vi "Check Mouse.vi"(7 "Packed refs":T1, 8 "error in (no error)":errorcluster, 11 "Board Game in":refnum<class "Board Game.lvclass">) -> (0 "error out":errorcluster, 3 "Board Game out":refnum<class "Board Game.lvclass">)   [LabVIEW 2021, in "Board Game.lvclass"]
uses:
  Board Game.lvclass
  Application/Packed Refs.ctl
  GameEl_class/private/Enum Direction.ctl
  LVApp/Modules/Sound Manager/Typedefs/Sound Effects.ctl
  Board Game.lvclass/Board Game.ctl
  GameEl_class/GameEl.lvclass/GameEl.ctl
  Mouse/Mouse.lvclass/Mouse.ctl
  <vilib>/numeric/Random Number (Range) U64.vi
  GameEl_class/Write Visible.vi
  Mouse/Write Init Mouse.vi
  Snake_class/Read Snake Head.vi
  GameEl_class/Read Visible.vi
  GameEl_class/Read position.vi
  <vilib>/numeric/sub_Random U32.vi
  Mouse/Mouse.lvclass
  C:/Users/poche/Programs/LabVIEW/imposible snake/GameEl_class/GameEl.lvclass
  Snake_class/Snake.lvclass
  GameEl_class/GameEl.lvclass
  Application/Application.lvclass
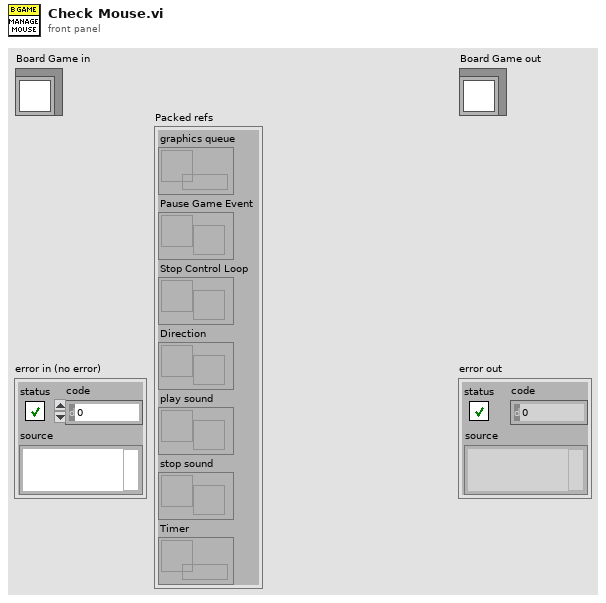
[diagram p1: front panel]
types:
  T1 = typedef "Application.lvclass/Packed Refs.ctl" = cluster{"graphics queue":refnum<queue>, "Pause Game Event":refnum<user-event>, "Stop Control Loop":refnum<user-event>, "Direction":refnum<notifier>, "play sound":refnum<user-event>, "stop sound":refnum<user-event>, "Timer":refnum<data-value>}
  T2 = typedef "Sound Effects.ctl" = enum16{"Bomb In", "Bomb Out", "Bomb Touched", "Game Over", "Victory", "Eat", "10 Fruits", "Eat2", "Eat3", "Eat4", "MaxShield", "Shield", "10p", "Grape In", "Grape Out", "20p", "30p", "40p", "50p", "60p", "70p", "80p", "90p", "100p", "All shields cracked", "Mouse In", "Mouse Out", "Mouse Eaten", "Grape Eaten", "States Recover", "Broken Shield", "Bonus", "Happy Time", "explode", "Game over musica", "Back Music", "Shield Catch", "Evil lough", "Cricket In", "Cricket eaten", "Lets Go", "Jump1", "Jump2", "Jump3", "Unstoppable", "Troll Music", "winner"}
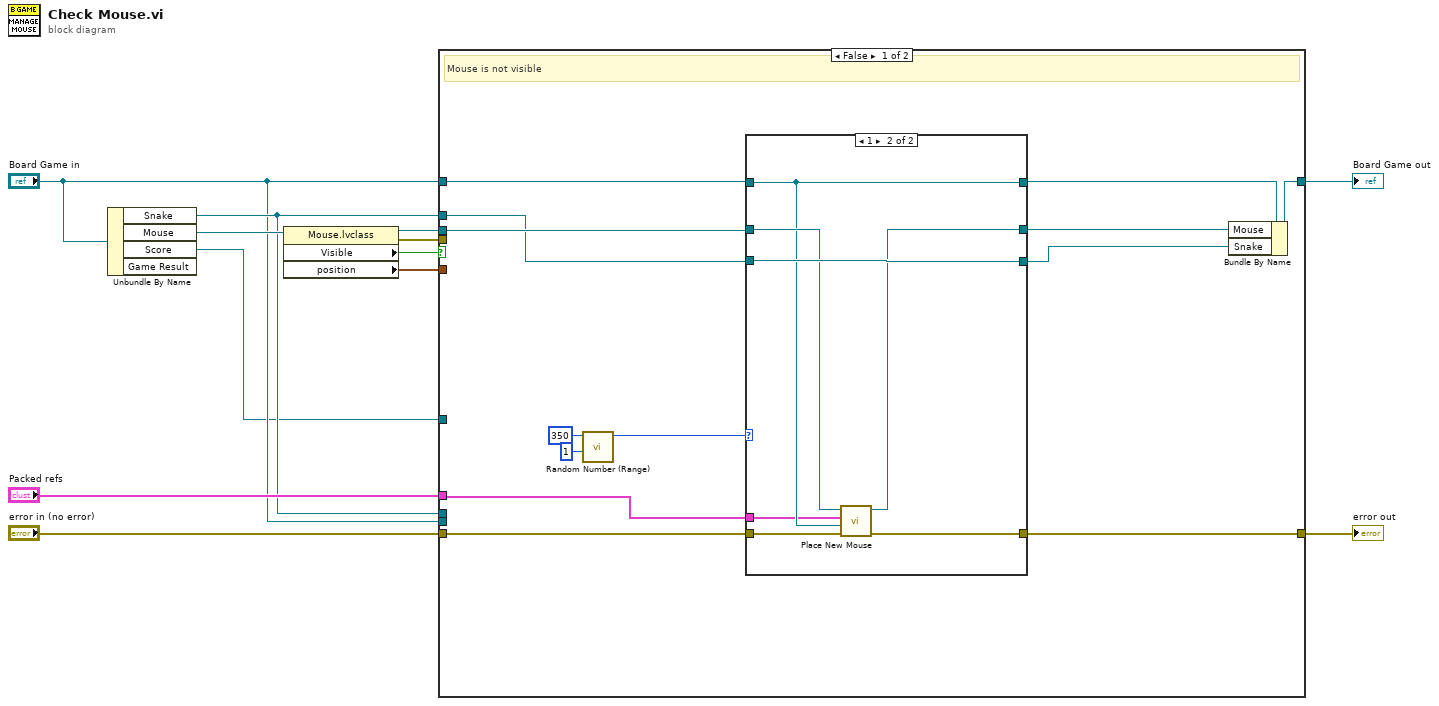
[diagram p0: block diagram]
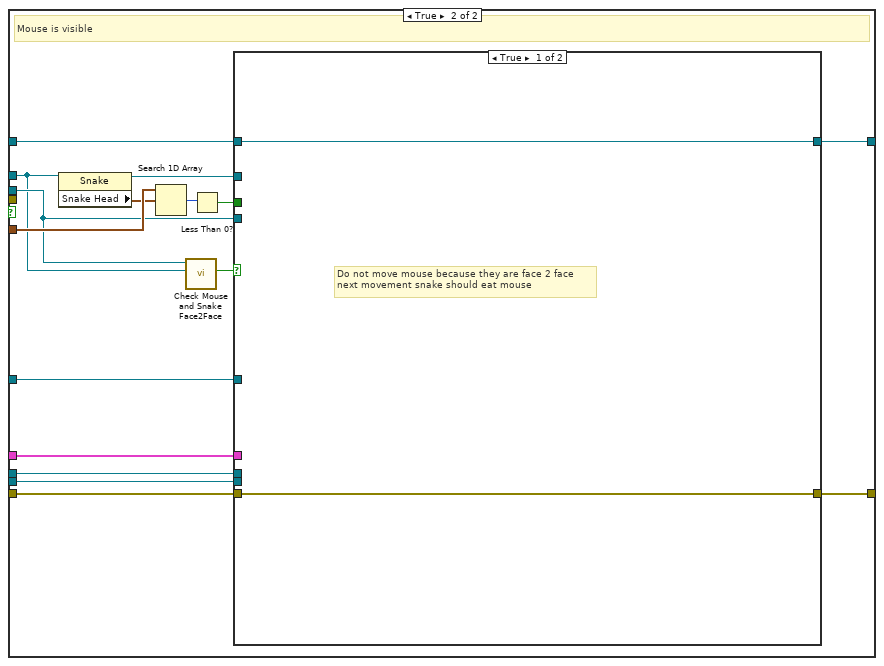
[diagram p3: hidden frame]
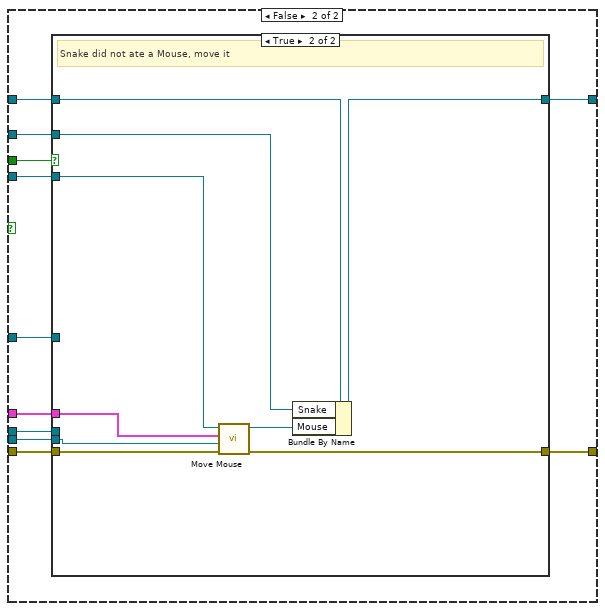
[diagram p4: hidden frame]
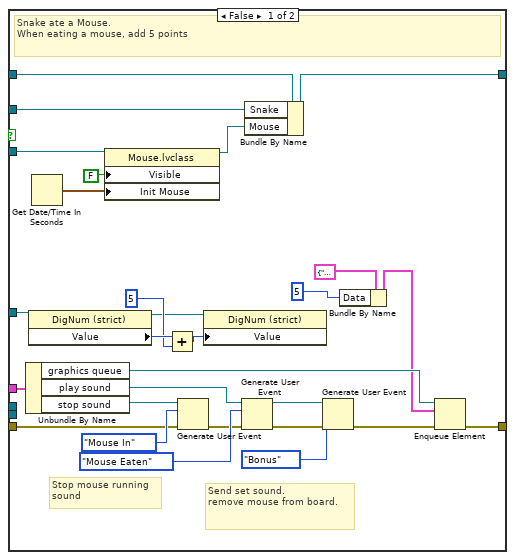
[diagram p5: hidden frame]
diagram:
  n1 = Unbundle By Name("Board Game in") -> ("Snake"=w4:refnum<class "Snake.lvclass">, "Mouse"=w12:refnum<class "Mouse.lvclass">, "Score"=w2:refnum<vi>)  [unwired: 1 out]
  n2 = property class="Mouse.lvclass"(reference=w12) -> (reference out=w9:refnum<class "Mouse.lvclass">, error out=w7:errorcluster, "Visible"=w10:bool, "position"=w8:cluster{"x":dbl, "y":dbl}[])  [unwired: 1 in]
  n3 = case shown="False" w10 {
    tunnel: "error in (no error)" -> [w23 w49]
    tunnel: "Board Game in" -> [w25 w47]
    tunnel: [w20 w46] -> w6
    tunnel: [w22 w48] -> w1
    tunnel: w9 -> [w21 w39]
    tunnel: w4 -> [w14 w38]
    tunnel: w8 -> [_ w52]
    tunnel: w7 -> [_ _]
    tunnel: "Packed refs" -> [w13 w43]
    tunnel: w4 -> [_ w42]
    tunnel: "Board Game in" -> [_ w41]
    tunnel: w2 -> [_ w40]
    frame False {
      # "Mouse is not visible"
      n4 = call-poly <vilib>:"Random Number (Range).vi"("lower bound (0)"=u64 1, "upper bound (100)"=u64 350) -> ("number"=w15:u64)  [unwired: 9 in]
      n5 = case shown="1" w15 {
        tunnel: w25 -> [w29 w31]
        tunnel: [w29 w31] -> w24
        tunnel: w23 -> [w28 w32]
        tunnel: [w28 w33] -> w22
        tunnel: w21 -> [w27 w35]
        tunnel: [w27 w34] -> w19
        tunnel: w14 -> [w26 w36]
        tunnel: [w26 w36] -> w18
        tunnel: w13 -> [_ w30]
        frame 0, Default {
        }
        frame 1 {
          n6 = call "Place New Mouse.vi"("error in (no error)"=w32, "Board Game in"=w31, "Packed refs"=w30, "Mouse in"=w35) -> ("error out"=w33:errorcluster, "Mouse out"=w34:refnum<class "Mouse.lvclass">)  [unwired: 6 in]
        }
      }
      n7 = Bundle By Name(cluster=w24, "Mouse"=w19, "Snake"=w18) -> (w20:refnum<class "Board Game.lvclass">)
    }
    frame True {
      # "Mouse is visible"
      n8 = property class="Snake"(reference=w38) -> (reference out=w44:refnum<class "Snake.lvclass">, "Snake Head"=w51:cluster{"x":dbl, "y":dbl})  [unwired: 1 in, 1 out]
      n9 = Search 1D Array(1D array=w52, element=w51) -> (index of element=w50:i32)  [unwired: 1 in]
      n10 = call "Check Mouse and Snake Face2Face.vi"("reference"=w38, "Mouse in"=w39) -> ("face 2 face?"=w37:bool)  [unwired: 7 in, 2 out]
      n11 = Less Than 0?(x=w50) -> (x < 0?=w45:bool)
      n12 = case shown="True" w37 {
        tunnel: w49 -> [w53 w65]
        tunnel: [w53 w64] -> w48
        tunnel: w47 -> [w54 w63]
        tunnel: [w54 w62] -> w46
        tunnel: w45 -> [_ w61]
        tunnel: w44 -> [_ w60]
        tunnel: w43 -> [_ w59]
        tunnel: w42 -> [_ w58]
        tunnel: w41 -> [_ w57]
        tunnel: w40 -> [_ w56]
        tunnel: w39 -> [_ w55]
        frame True {
          # "Do not move mouse because they are face 2 face\nnext movement snake should eat mouse"
        }
        frame False {
          n13 = case shown="True" w61 {
            tunnel: w65 -> [w77 w99]
            tunnel: [w74 w98] -> w64
            tunnel: w63 -> [w93 w102]
            tunnel: [w92 w101] -> w62
            tunnel: w55 -> [w91 w96]
            tunnel: w60 -> [w88 w100]
            tunnel: w59 -> [w82 w94]
            tunnel: w58 -> [_ _]
            tunnel: w57 -> [_ w95]
            tunnel: w56 -> [w87 _]
            frame False {
              # "Stop mouse running\nsound"
              # "Send set sound.\nremove mouse from board."
              # "Snake ate a Mouse. \nWhen eating a mouse, add 5 points"
              n14 = Unbundle By Name(w82) -> ("graphics queue"=w73:refnum<queue>, "play sound"=w79:refnum<user-event>, "stop sound"=w75:refnum<user-event>)
              n15 = property class="DigNum (strict)"(reference=w87) -> (reference out=w83:refnum<vi>, "Value"=w86:u16)  [unwired: 1 in, 1 out]
              n16 = Get Date/Time In Seconds() -> (seconds since 1Jan1904=w81:timestamp)
              n17 = property class="Mouse.lvclass"(reference=w91, "Visible"=FALSE, "Init Mouse"=w81) -> (reference out=w90:refnum<class "Mouse.lvclass">)  [unwired: 1 in, 1 out]
              n18 = Add(x=w86, y=u16 5) -> (x+y=w84:u16)
              n19 = Generate User Event(user event=w75, event data cluster=Sound_Effects."Mouse In" ("event data"), error in=w77) -> (error out=w76:errorcluster)  [unwired: 1 in, 1 out]
              n20 = property class="DigNum (strict)"(reference=w83, "Value"=w84) -> ()  [unwired: 1 in, 2 out]
              n21 = Generate User Event(user event=w79, event data cluster=Sound_Effects."Mouse Eaten" ("event data"), error in=w76) -> (user event out=w69:refnum<user-event>, error out=w67:errorcluster)  [unwired: 1 in]
              n22 = Bundle By Name(cluster=w93, "Snake"=w88, "Mouse"=w90) -> (w92:refnum<class "Board Game.lvclass">)
              n23 = Generate User Event(user event=w69, event data cluster=Sound_Effects."Bonus" ("event data"), error in=w67) -> (error out=w66:errorcluster)  [unwired: 1 in, 1 out]
              n24 = Bundle By Name(cluster=cluster{"Message":string, "Data":variant} {"Message"="10 Points", "Data"=variant} ("element"), "Data"=u16 5) -> (w71:cluster{"Message":string, "Data":variant})
              n25 = Enqueue Element(queue=w73, element=w71, error in (no error)=w66) -> (error out=w74:errorcluster)  [unwired: 1 in, 2 out]
            }
            frame True {
              # "Snake did not ate a Mouse, move it"
              n26 = call "Move Mouse.vi"("error in (no error)"=w99, "Board Game in"=w95, "Packed refs"=w94, "Mouse in"=w96) -> ("error out"=w98:errorcluster, "Mouse out"=w97:refnum<class "Mouse.lvclass">)  [unwired: 6 in]
              n27 = Bundle By Name(cluster=w102, "Snake"=w100, "Mouse"=w97) -> (w101:refnum<class "Board Game.lvclass">)
            }
          }
        }
      }
    }
  }
  "error out" <- w1
  "Board Game out" <- w6
